vi "Raise Source Changed Event.vi"(4 "Event in":refnum<user-event>, 5 "Event Data":cluster{"sender":refnum<k24>, "e":refnum<k24>}, 6 "Control Ref":refnum<k24>, 7 "Event Common Data":T1) -> ()   [LabVIEW 2024, in "WebView.lvclass"]
uses:
  WebView.lvclass
  <vilib>/sklein/WebView2/Libs/Microsoft.Web.WebView2.Core.dll
  Source Changed Event Data--cluster.ctl
  WebView.lvclass/WebView.ctl
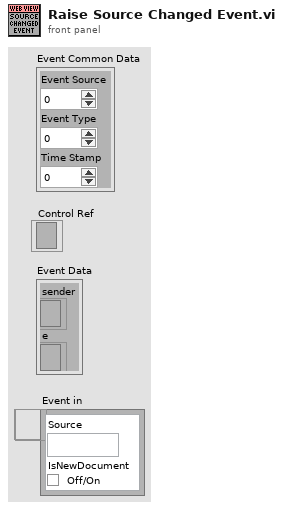
[diagram p1: front panel]
types:
  T1 = cluster{"Event Source":i32, "Event Type":u32, "Time Stamp":u32}
  T2 = typedef "WebView.lvclass/Source Changed Event Data--cluster.ctl" = cluster{"Source":string, "IsNewDocument":bool}
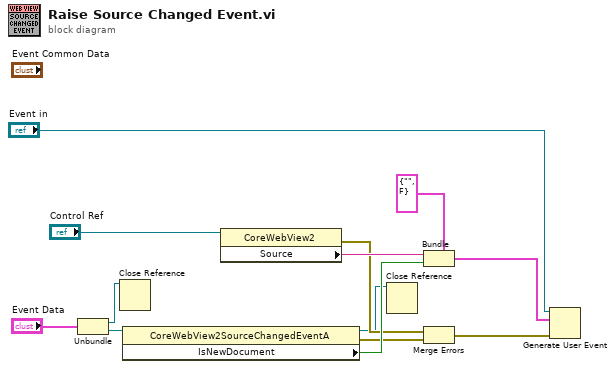
[diagram p0: block diagram]
diagram:
  n1 = Unbundle("Event Data") -> ("sender"=w4:refnum<k24>, "e"=w12:refnum<k24>)
  n2 = Close Reference(reference=w4) -> ()  [unwired: 1 in, 1 out]
  n3 = property class="CoreWebView2SourceChangedEventA"(reference=w12) -> (reference out=w3:refnum<k24>, error out=w7:errorcluster, "IsNewDocument"=w10:bool)  [unwired: 1 in]
  n4 = property class="CoreWebView2"(reference="Control Ref") -> (error out=w5:errorcluster, "Source"=w9:string)  [unwired: 1 in, 1 out]
  n5 = Close Reference(reference=w3) -> ()  [unwired: 1 in, 1 out]
  n6 = Bundle(cluster=T2 {"Source"="", "IsNewDocument"=FALSE} ("Source"), "Source"=w9, "IsNewDocument"=w10) -> (w8:T2)
  n7 = Merge Errors(w5, w7) -> (w6:errorcluster)
  n8 = Generate User Event(user event="Event in", event data cluster=w8, error in=w6) -> ()  [unwired: 1 in, 2 out]
